vi "NI VeriStand - Generate cRIO FPGA Clock.vi"(9 "Use External Timing":bool, 10 "Write to  RTSI":bool, 11 "Loop Rate (usec)":u32) -> ()   [LabVIEW 2010, in "NI_VS FPGA Clock Support.lvlib"]
uses:
  <userlib>/_NI VeriStand FPGA Support/NI VeriStand FPGA Clock Support/NI_VS FPGA Clock Support.lvlib
  <userlib>/_NI VeriStand FPGA Support/NI VeriStand FPGA Clock Support/NI VeriStand - Timing Engine Globals.vi
  <vilib>/eio/EIOMethodNode/EIOMethodNode.xnode
  <vilib>/eio/EIONode/EIONode.xnode
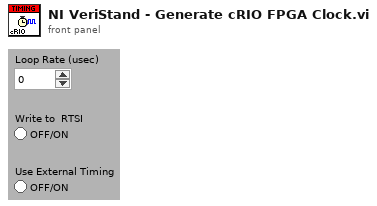
[diagram p1: front panel]
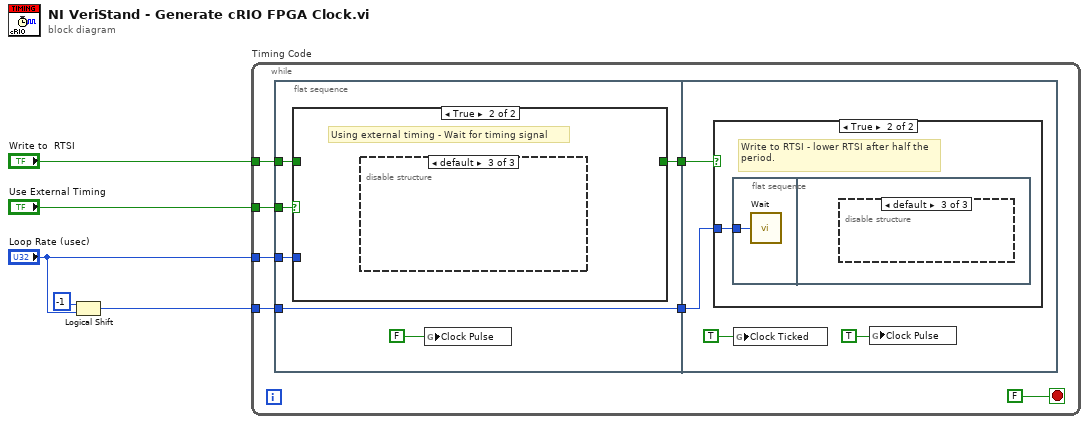
[diagram p0: block diagram]
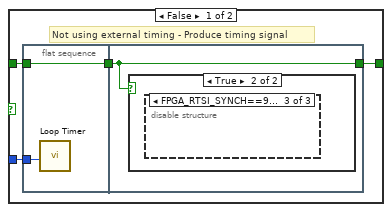
[diagram p2: hidden frame]
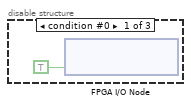
[diagram p4: hidden frame]
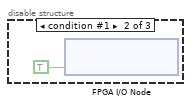
[diagram p5: hidden frame]
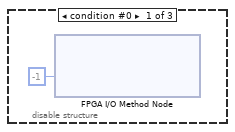
[diagram p6: hidden frame]
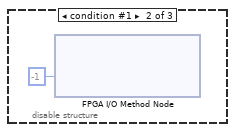
[diagram p7: hidden frame]
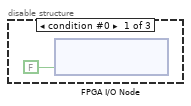
[diagram p9: hidden frame]
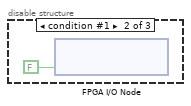
[diagram p10: hidden frame]
diagram:
  n1 = Logical Shift(y=i8 -1, x="Loop Rate (usec)") -> (x << y=w2:u32)
  n2 = while "Timing Code" {
    tunnel: w2 -> [w12]
    tunnel: "Loop Rate (usec)" -> [w11]
    tunnel: "Use External Timing" -> [w10]
    tunnel: "Write to  RTSI" -> [w9]
    stop <- FALSE stop-if-true
    n3 = flat-sequence {
      tunnel: w12 -> [w15]
      tunnel: w11 -> [w18]
      tunnel: w10 -> [w17]
      tunnel: w9 -> [w16]
      tunnel: [w15] -> w7
      tunnel: [w14] -> w6
      tunnel: w7 -> [w37]
      tunnel: w6 -> [w36]
      frame #0 {
        n4 = case shown="True" w17 {
          tunnel: w18 -> [w22 _]
          tunnel: w16 -> [w20 _]
          tunnel: [w19 _] -> w14
          frame False {
            # "Not using external timing - Produce timing signal"
            n5 = flat-sequence {
              tunnel: [w23] -> w21
              tunnel: w22 -> [w24]
              tunnel: w20 -> [w23]
              tunnel: w21 -> [w25]
              tunnel: [w25] -> w19
              frame #0 {
                n6 = call "Loop Timer"("Count(uSec)"=w24) -> ()  [unwired: 1 out]
              }
              frame #1 {
                n7 = case shown="True" w25 {
                  frame False {
                  }
                  frame True {
                    n8 = disable-structure shown="FPGA_RTSI_SYNCH==9402" {
                      frame condition #0 {
                        n9 = xnode "FPGA I/O Node"("NI 9401/DIO0"=TRUE ("TRIG0")) -> ()  [unwired: 1 in, 1 out]
                      }
                      frame condition #1 {
                        n10 = xnode "FPGA I/O Node"("NI 9402/DIO0"=TRUE ("TRIG0")) -> ()  [unwired: 1 in, 1 out]
                      }
                      frame condition #2 (active) {
                      }
                    }
                  }
                }
              }
            }
          }
          frame True {
            # "Using external timing - Wait for timing signal"
            n11 = disable-structure shown="default" {
              frame condition #0 {
                n12 = xnode "FPGA I/O Method Node"("Timeout"=-1) -> ()  [unwired: 1 in, 2 out]
              }
              frame condition #1 {
                n13 = xnode "FPGA I/O Method Node"("Timeout"=-1) -> ()  [unwired: 1 in, 2 out]
              }
              frame condition #2 (active) {
              }
            }
          }
        }
        n14 = global write "NI VeriStand - Timing Engine Globals.vi" "Clock Pulse"(FALSE ("Clock Ticked")) -> ()
      }
      frame #1 {
        n15 = case shown="True" w36 {
          tunnel: w37 -> [_ w38]
          frame False {
          }
          frame True {
            # "Write to RTSI - lower RTSI after half the period."
            n16 = flat-sequence {
              tunnel: w38 -> [w39]
              frame #0 {
                n17 = call "Wait"("Count(uSec)"=w39) -> ()  [unwired: 1 out]
              }
              frame #1 {
                n18 = disable-structure shown="default" {
                  frame condition #0 {
                    n19 = xnode "FPGA I/O Node"("NI 9401/DIO0"=FALSE ("TRIG0")) -> ()  [unwired: 1 in, 1 out]
                  }
                  frame condition #1 {
                    n20 = xnode "FPGA I/O Node"("NI 9402/DIO0"=FALSE ("TRIG0")) -> ()  [unwired: 1 in, 1 out]
                  }
                  frame condition #2 (active) {
                  }
                }
              }
            }
          }
        }
        n21 = global write "NI VeriStand - Timing Engine Globals.vi" "Clock Ticked"(TRUE ("Clock Ticked")) -> ()
        n22 = global write "NI VeriStand - Timing Engine Globals.vi" "Clock Pulse"(TRUE ("Clock Ticked")) -> ()
      }
    }
  }
